vi "main.vi"() -> ()   [LabVIEW 2020]
doc: "This VI is used as the driver for the queue to work. It performs the operations in the queue."
uses:
  Typedef's/Data_Cluster.ctl
  Typedef's/Content_Level.ctl
  Typedef's/Bewarage_Out_Level.ctl
  Typedef's/Timer_Details.ctl
  Typedef's/Timings_Map.ctl
  Typedef's/Operation_Indication.ctl
  Typedef's/Low_Level_Indications.ctl
  Typedef's/Q_Operations.ctl
  <vilib>/Utility/error.llb/DialogType.ctl
  <vilib>/Utility/config.llb/Read Key (Boolean).vi
  <vilib>/Utility/config.llb/Read Key (I32).vi
  <vilib>/Utility/config.llb/Read Key (U32).vi
  <vilib>/Utility/config.llb/Write Key (U32).vi
  <vilib>/Utility/config.llb/Write Key (I32).vi
  <vilib>/Utility/config.llb/NI_LVConfig.lvlib
panel:
  in  "Error In":errorcluster
  in  "Power":bool
  out "Total Cups":u32
  out "Elapsed Time":i32
  out "Dispensing":bool
  out "Brewing":bool
  out "Grinding":bool
  out "Heating":bool
  out "Purging":bool
  in  "Dispenser":dbl(slide) min=-0.0 max=60.0 step=1.0 scale=0.0..60.0
  in  "Chamber":dbl(slide) min=-0.0 max=60.0 step=1.0 scale=0.0..60.0
  out "Low Milk":bool
  out "Low Bean":bool
  out "Low Water":bool
  out "Milk Level":i32(slide) min=0 max=100 step=1 scale=0.0..100.0
  out "Bean Level":i32(slide) min=0 max=100 step=1 scale=0.0..100.0
  out "Water Level":i32(slide) min=0 max=100 step=1 scale=0.0..100.0
  in  "Bewarage":i32(knob) min=0 max=2 step=1 scale=0.0..2.0
  in  "Carafe":bool
  in  "1 Cup":bool
  # "Description: \n-> Only after power run. Make the button press\nto make coffee"
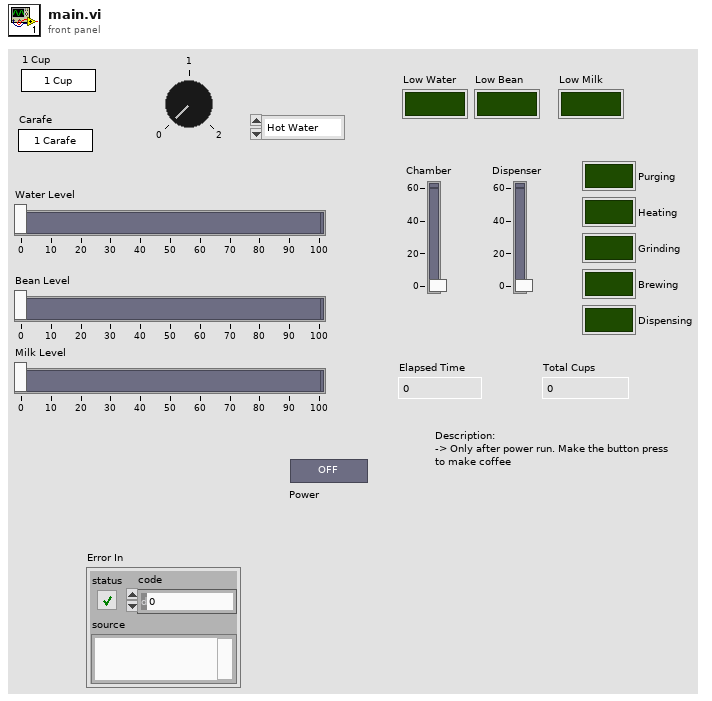
[diagram p1: front panel]
types:
  T1 = typedef "Q_Operations.ctl" = enum16{"Create Q", "Enqueue ", "Dequeue", "Enqueue N ele", "Enstack N ele", "Flush Q", "Destroy Q"}
  T2 = typedef "Data_Cluster.ctl" = cluster{"Cup":bool, "Bewarage":dbl, "Carafe":bool, "Power":bool, "Content Levels":T3, "Beware Out Level":T4, "Data File path":path, "Timer Operations":T5, "Cups Count":u32, "Bewarage Low Level":i32, "Timings Map":T6, "Sequence Array":string[], "Operation Indication":T7, "Bewarage Selection":string, "Low Level Indications":T8}
  T3 = typedef "Content_Level.ctl" = cluster{"Water Level":i32, "Bean Level":i32, "Milk Level":i32}
  T4 = typedef "Bewarage_Out_Level.ctl" = cluster{"Dispenser":dbl, "Chamber":dbl}
  T5 = typedef "Timer_Details.ctl" = cluster{"Set Time":dbl, "Prev Time":dbl, "Elapsed Time":dbl, "Start?":bool, "Paused?":bool}
  T6 = typedef "Timings_Map.ctl" = cluster{"Operation map":map{string, i32}, "Bevarage Timings":map{string, i32}}
  T7 = typedef "Operation_Indication.ctl" = cluster{"Heating":bool, "Grinding":bool, "Dispensing":bool, "Purging":bool, "Brewing":bool}
  T8 = typedef "Low_Level_Indications.ctl" = cluster{"Low Water":bool, "Low Milk":bool, "Low Bean":bool}
  T9 = typedef "NI_LVConfig.lvlib/Config Data RefNum.ctl" = refnum<k1>
  T10 = typedef "DialogType.ctl" = u16
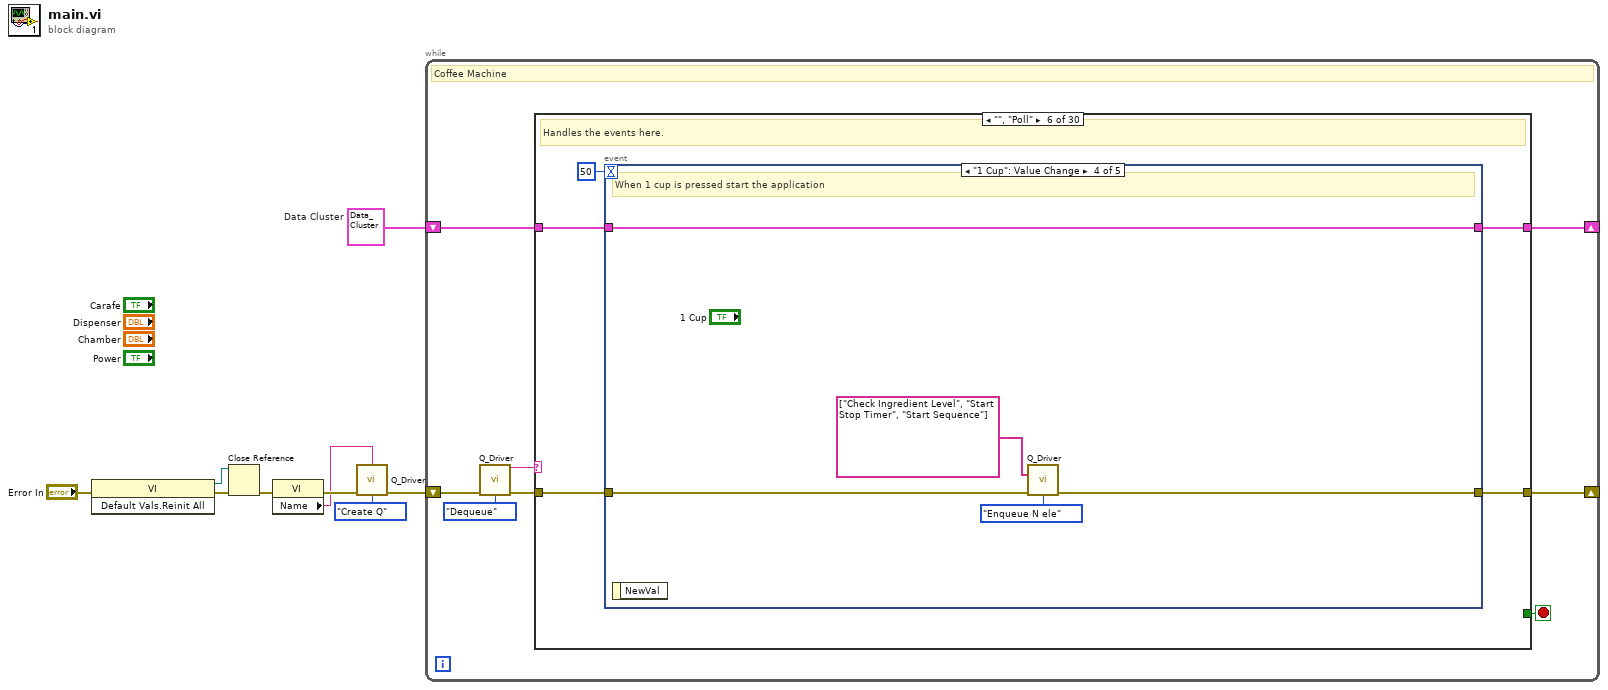
[diagram p0: block diagram]
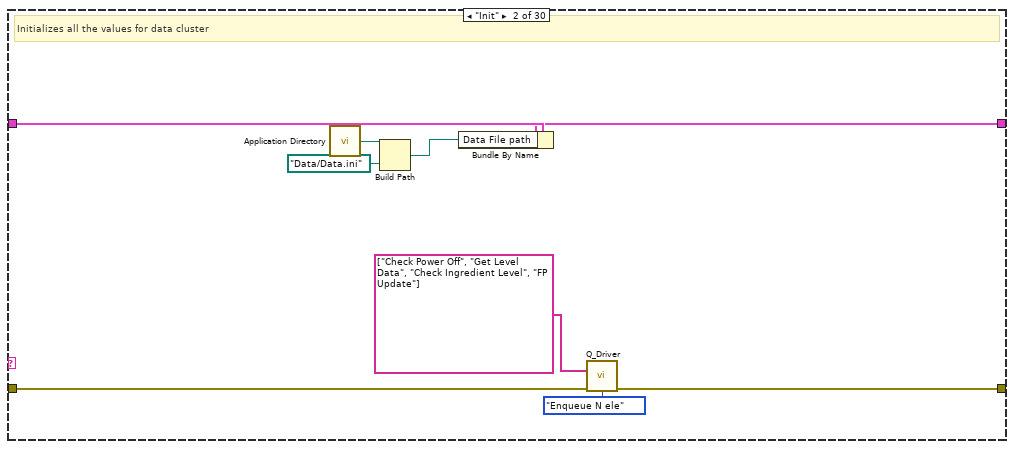
[diagram p3: hidden frame]
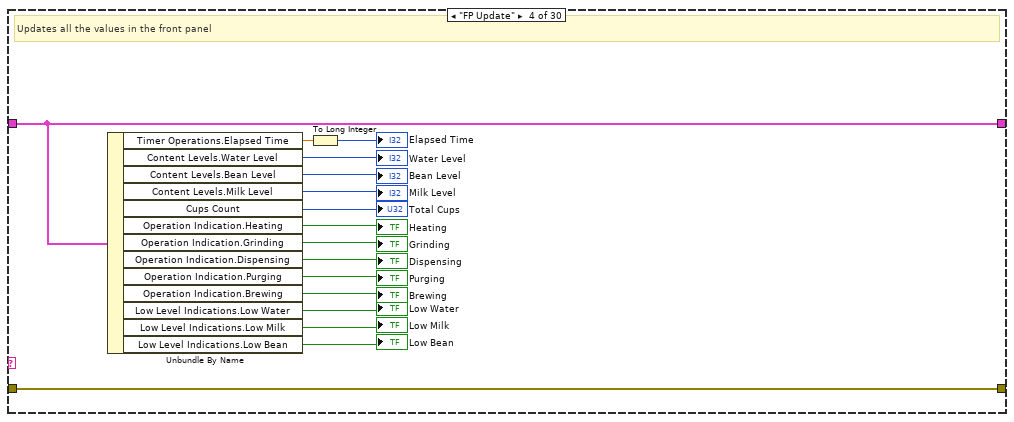
[diagram p5: hidden frame]
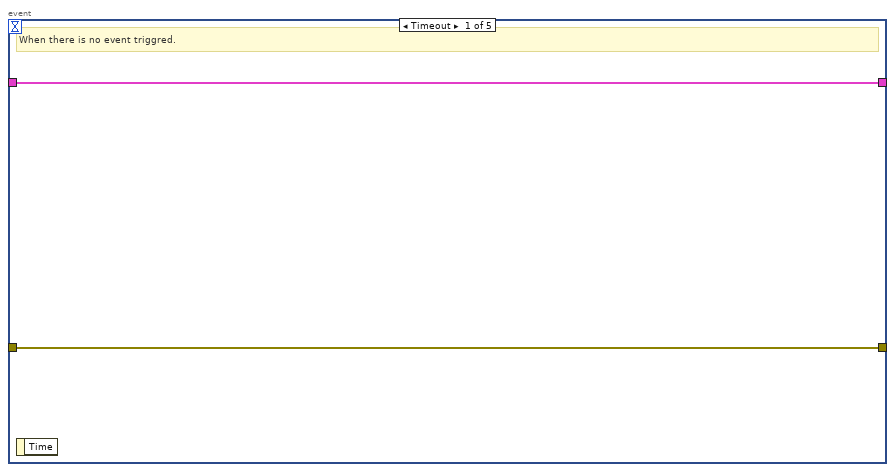
[diagram p7: hidden frame]
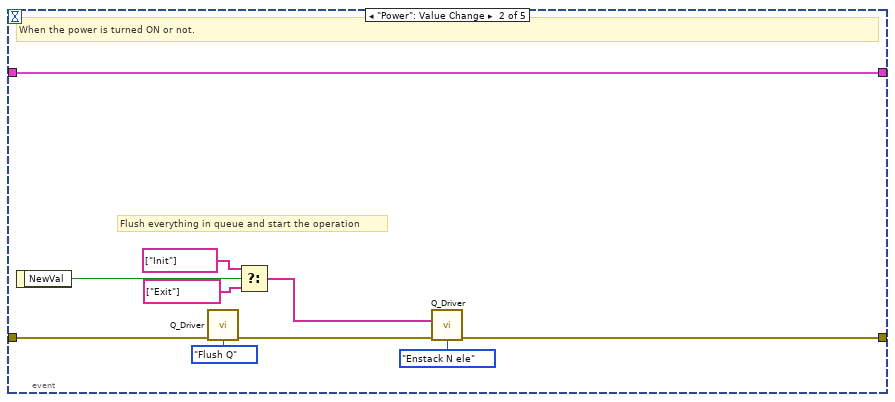
[diagram p8: hidden frame]
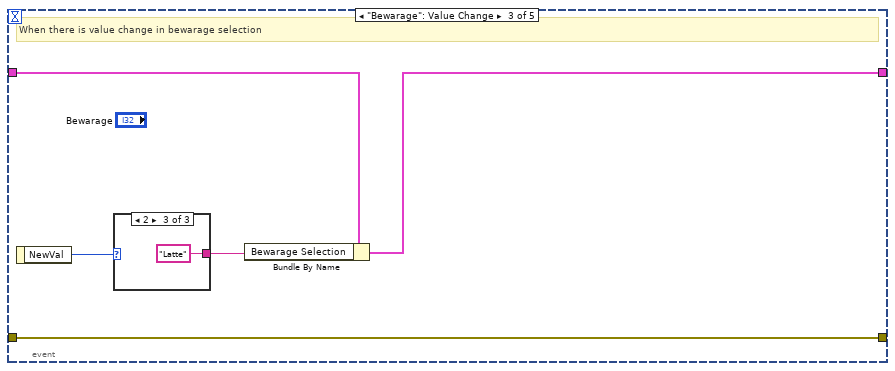
[diagram p9: hidden frame]
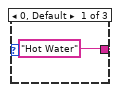
[diagram p10: hidden frame]
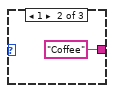
[diagram p11: hidden frame]
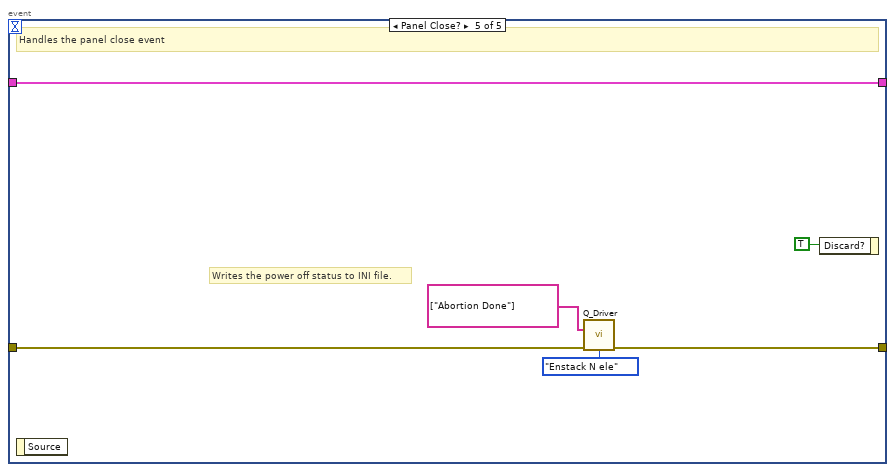
[diagram p12: hidden frame]
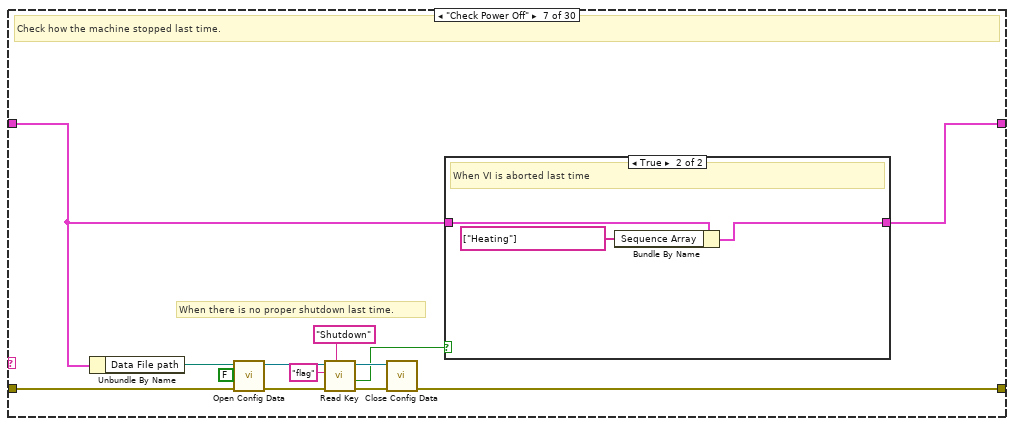
[diagram p13: hidden frame]
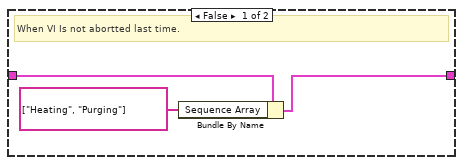
[diagram p14: hidden frame]
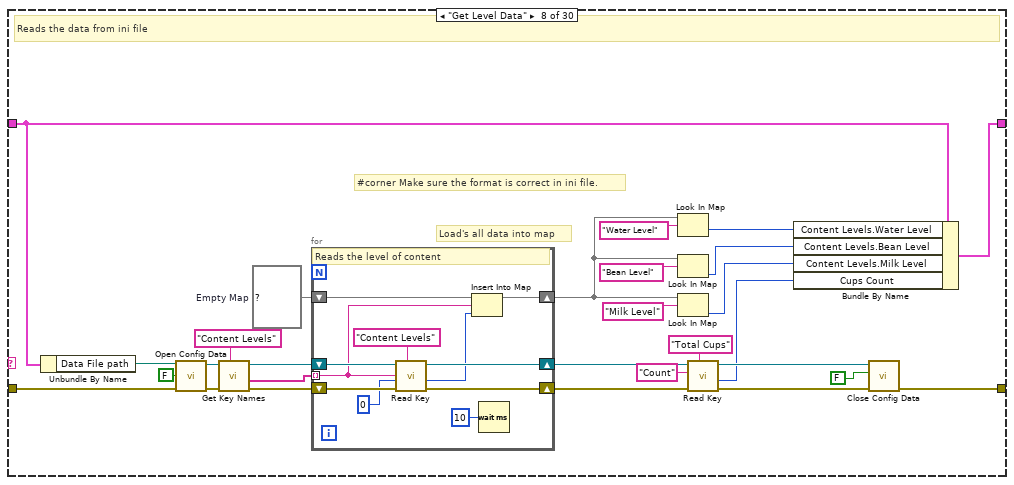
[diagram p15: hidden frame]
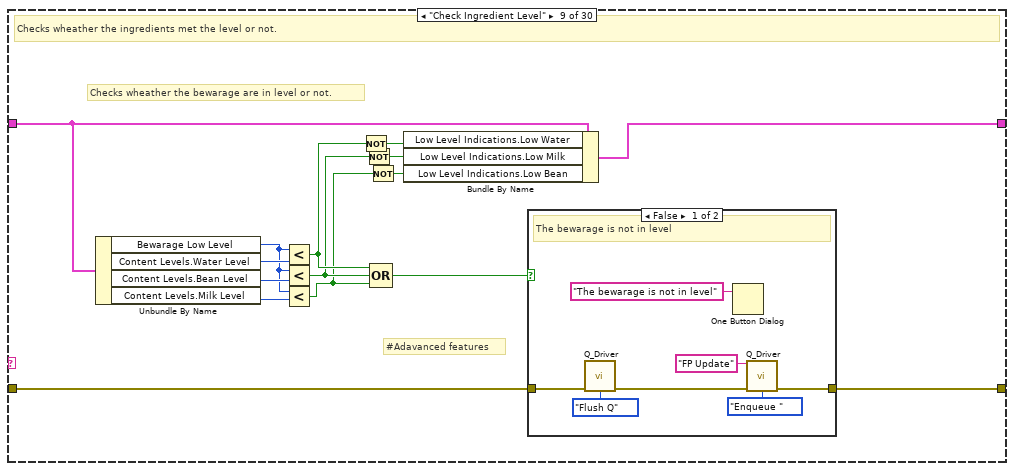
[diagram p16: hidden frame]
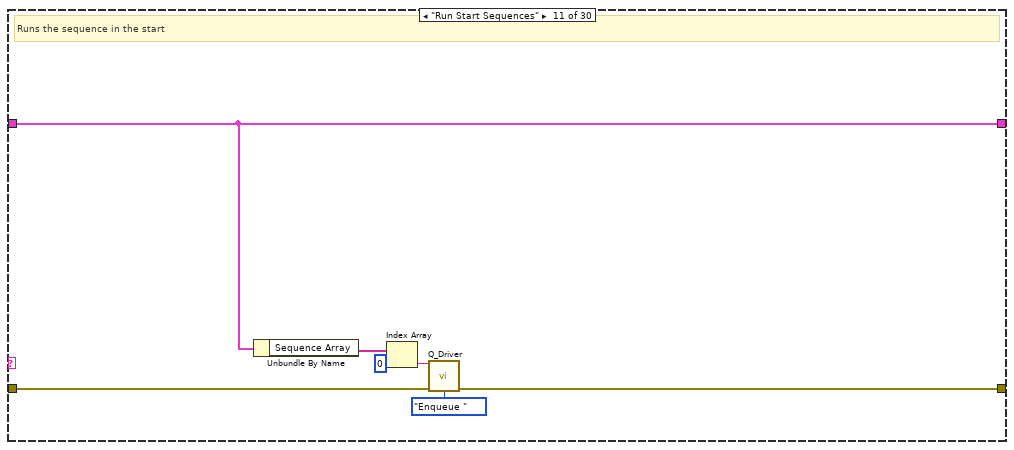
[diagram p19: hidden frame]
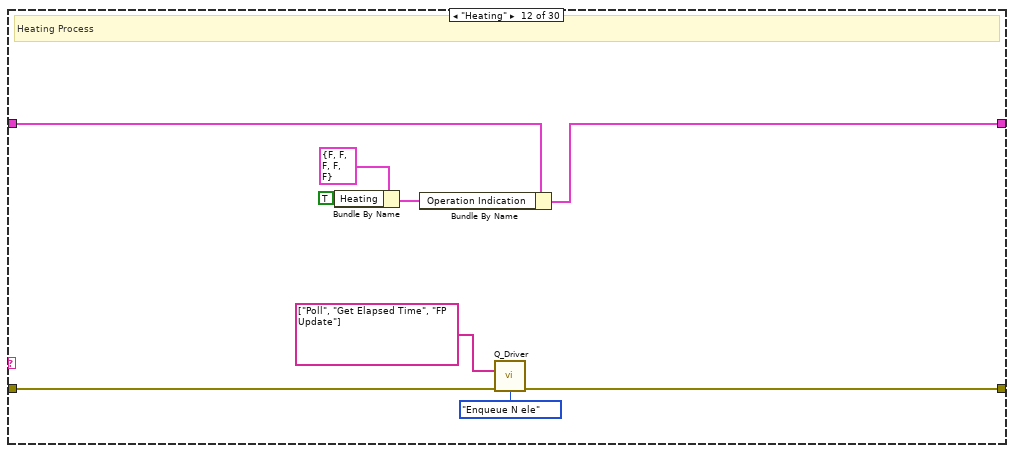
[diagram p20: hidden frame]
diagram:
  w4 = T2 {"Cup"=FALSE, "Bewarage"=0.0, "Carafe"=FALSE, "Power"=FALSE, "Content Levels"={"Water Level"=0, "Bean Level"=0, "Milk Level"=0}, "Beware Out Level"={"Dispenser"=0.0, "Chamber"=0.0}, "Data File path"=path "", "Timer Operations"={"Set Time"=0.0, "Prev Time"=0.0, "Elapsed Time"=0.0, "Start?"=FALSE, "Paused?"=FALSE}, "Cups Count"=0, "Bewarage Low Level"=30, "Timings Map"={"Operation map"={"Heating"=5, "Purging"=4}, "Bevarage Timings"={"Brewing"=4, "Dispensing"=5, "Grinding"=3}}, "Sequence Array"=[], "Operation Indication"={"Heating"=FALSE, "Grinding"=FALSE, "Dispensing"=FALSE, "Purging"=FALSE, "Brewing"=FALSE}, "Bewarage Selection"="Hot Water", "Low Level Indications"={"Low Water"=FALSE, "Low Milk"=FALSE, "Low Bean"=FALSE}}  # Data Cluster
  n1 = invoke class="VI" method="Default Vals.Reinit All"(error in="Error In") -> (reference out=w1:refnum<vi>, error out=w3:errorcluster)  [unwired: 2 in, 1 out]
  n2 = Close Reference(reference=w1, error in (no error)=w3) -> (error out=w2:errorcluster)
  n3 = property class="VI"(error in=w2) -> (error out=w6:errorcluster, "Name"=w5:string)  [unwired: 1 in, 1 out]
  n4 = call "Q_Driver.vi"("Q Name"=w5, "Error In"=w6, "Operations"=Q_Operations."Create Q") -> ("Error Out"=w8:errorcluster)  [unwired: 11 in, 1 out]
  n5 = while {
    shift-right: [w16] -> _
    shift-left: w8 -> [w17]
    shift-right: [w11] -> _
    shift-left: w4 -> [w12]
    stop <- w10 stop-if-true
    # "Coffee Machine"
    n6 = call "Q_Driver.vi"("Error In"=w17, "Operations"=Q_Operations."Dequeue") -> ("Dequeued Ele"=w13:string, "Error Out"=w15:errorcluster)  [unwired: 12 in]
    n7 = case shown="\"\", \"Poll\"" w13 {
      tunnel: w15 -> [w19 w27 w30 w46 w48 w53 w97 w131 w147 w167 w174 w183 w192 w194 w201 w240 w249 w250 w259 w276 w320 w322 w331 w342 w361 w367 w369 w375 w381 w383]
      tunnel: [w19 w26 w30 w46 w48 w52 w95 w128 w146 w167 w170 w181 w190 w194 w197 w239 w243 w251 w260 w271 w287 w322 w331 w333 w361 w364 w369 w372 w379 w383] -> w16
      tunnel: w12 -> [w18 w28 w29 w45 w47 w50 w86 w111 w157 w166 w173 w182 w191 w193 w199 w238 w248 w258 w263 w274 w315 w321 w329 w341 w360 w362 w368 w374 w378 w382]
      tunnel: [w18 w21 w29 w45 w47 w49 w85 w115 w151 w166 w173 w178 w187 w193 w198 w232 w247 w255 w264 w275 w305 w321 w330 w337 w360 w362 w368 w374 w378 w382] -> w11
      tunnel: [_ _ _ _ _ _ _ _ _ _ _ _ _ _ _ _ _ _ _ _ _ _ _ _ _ _ _ TRUE TRUE _] -> w10
      frame "/**** Initialization ****/" {
      }
      frame "Init" {
        # "Initializes all the values for data cluster"
        n8 = call <vilib>:"Application Directory.vi"() -> ("Application Directory"=w23:path)
        n9 = Build Path(base path=w23, name or relative path=path "Data/Data.ini") -> (appended path=w20:path)
        n10 = Bundle By Name(cluster=w28, "Data File path"=w20) -> (w21:T2)
        n11 = call "Q_Driver.vi"("States[]"=string[] ["Check Power Off", "Get Level Data", "Check Ingredient Level", "FP Update"], "Error In"=w27, "Operations"=Q_Operations."Enqueue N ele") -> ("Error Out"=w26:errorcluster)  [unwired: 11 in, 1 out]
      }
      frame "/***** FP Related ****/" {
      }
      frame "FP Update" {
        # "Updates all the values in the front panel"
        n12 = Unbundle By Name(w45) -> ("Timer Operations.Elapsed Time"=w35:dbl, "Content Levels.Water Level"=→"Water Level":i32, "Content Levels.Bean Level"=→"Bean Level":i32, "Content Levels.Milk Level"=→"Milk Level":i32, "Cups Count"=→"Total Cups":u32, "Operation Indication.Heating"=→"Heating":bool, "Operation Indication.Grinding"=→"Grinding":bool, "Operation Indication.Dispensing"=→"Dispensing":bool, "Operation Indication.Purging"=→"Purging":bool, "Operation Indication.Brewing"=→"Brewing":bool, "Low Level Indications.Low Water"=→"Low Water":bool, "Low Level Indications.Low Milk"=→"Low Milk":bool, "Low Level Indications.Low Bean"=→"Low Bean":bool)
        n13 = To Long Integer(number=w35) -> (32bit integer=→"Elapsed Time":i32)
      }
      frame "/***** Events and Functionalities *****/" {
      }
      frame "", "Poll" {
        # "Handles the events here."
        n14 = event shown="[3] \"1 Cup\": Value Change" {
          selector: _ -> [_ _ _ _ _]
          dyn-events: _ -> [_ _ _ _ _]
          timeout: 50 -> [_ _ _ _ _]
          tunnel: [w55 w60 w70 w76 w82] -> w52
          tunnel: w53 -> [w55 w65 w70 w78 w84]
          tunnel: [w54 w64 w67 w77 w79] -> w49
          tunnel: w50 -> [w54 w64 w69 w77 w79]
          event Timeout {
            # "When there is no event triggred."
            n15 = event-data() -> ()  [unwired: 1 in, 1 out]
          }
          event "Power": Value Change {
            # "Flush everything in queue and start the operation"
            # "When the power is turned ON or not."
            n16 = event-data() -> ("NewVal"=w63:bool)  [unwired: 1 in]
            n17 = call "Q_Driver.vi"("Error In"=w65, "Operations"=Q_Operations."Flush Q") -> ("Error Out"=w57:errorcluster)  [unwired: 12 in, 1 out]
            n18 = Select(t=string[] ["Init"], s=w63, f=string[] ["Exit"]) -> (s? t:f=w58:string[])
            n19 = call "Q_Driver.vi"("States[]"=w58, "Error In"=w57, "Operations"=Q_Operations."Enstack N ele") -> ("Error Out"=w60:errorcluster)  [unwired: 11 in, 1 out]
          }
          event "Bewarage": Value Change {
            # "When there is value change in bewarage selection"
            n20 = event-data() -> ("NewVal"=w68:i32)  [unwired: 1 in]
            n21 = case shown="2" w68 {
              tunnel: ["Hot Water" "Coffee" "Latte"] -> w66
              frame 0, Default {
              }
              frame 1 {
              }
              frame 2 {
              }
            }
            n22 = Bundle By Name(cluster=w69, "Bewarage Selection"=w66) -> (w67:T2)
          }
          event "1 Cup": Value Change {
            # "When 1 cup is pressed start the application"
            n23 = event-data() -> ()  [unwired: 1 in, 1 out]
            n24 = call "Q_Driver.vi"("States[]"=string[] ["Check Ingredient Level", "Start Stop Timer", "Start Sequence"], "Error In"=w78, "Operations"=Q_Operations."Enqueue N ele") -> ("Error Out"=w76:errorcluster)  [unwired: 11 in, 1 out]
          }
          event Panel Close? {
            # "Writes the power off status to INI file."
            # "Handles the panel close event"
            n25 = event-data() -> ()  [unwired: 1 in, 1 out]
            n26 = call "Q_Driver.vi"("States[]"=string[] ["Abortion Done"], "Error In"=w84, "Operations"=Q_Operations."Enstack N ele") -> ("Error Out"=w82:errorcluster)  [unwired: 11 in, 1 out]
            n27 = event-data("Discard?"=TRUE) -> ()  [unwired: 1 in, 1 out]
          }
        }
      }
      frame "Check Power Off" {
        # "When there is no proper shutdown last time."
        # "Check how the machine stopped last time."
        n28 = Unbundle By Name(w86) -> ("Data File path"=w88:path)
        n29 = call <vilib>:"Open Config Data.vi"("error in (no error)"=w97, "create file if necessary (T)"=FALSE, "configuration file path"=w88) -> ("error out"=w94:errorcluster, "refnum"=w93:T9)  [unwired: 6 in, 1 out]
        n30 = call-poly <vilib>:"Read Key.vi"("section"="Shutdown", "error in (no error)"=w94, "key"="flag", "refnum"=w93) -> ("error out"=w91:errorcluster, "value"=w87:bool, "refnum out"=w92:T9)  [unwired: 4 in, 1 out]
        n31 = call <vilib>:"Close Config Data.vi"("error in (no error)"=w91, "refnum"=w92) -> ("error out"=w95:errorcluster)  [unwired: 8 in, 1 out]
        n32 = case shown="True" w87 {
          tunnel: w86 -> [w100 w103]
          tunnel: [w99 w102] -> w85
          frame False {
            # "When VI Is not abortted last time."
            n33 = Bundle By Name(cluster=w100, "Sequence Array"=string[] ["Heating", "Purging"]) -> (w99:T2)
          }
          frame True {
            # "When VI is aborted last time"
            n34 = Bundle By Name(cluster=w103, "Sequence Array"=string[] ["Heating"]) -> (w102:T2)
          }
        }
      }
      frame "Get Level Data" {
        w121 = map{string, i32} {}  # Empty Map
        # "Load's all data into map"
        # "#corner Make sure the format is correct in ini file."
        # "Reads the data from ini file"
        n35 = Unbundle By Name(w111) -> ("Data File path"=w110:path)
        n36 = call <vilib>:"Open Config Data.vi"("error in (no error)"=w131, "create file if necessary (T)"=FALSE, "configuration file path"=w110) -> ("error out"=w129:errorcluster, "refnum"=w125:T9)  [unwired: 6 in, 1 out]
        n37 = call <vilib>:"Get Key Names.vi"("section"="Content Levels", "error in (no error)"=w129, "refnum"=w125) -> ("error out"=w126:errorcluster, "key names"=w123:string[], "refnum out"=w122:T9)  [unwired: 5 in, 1 out]
        n38 = for {
          shift-right: [w141] -> w124
          shift-left: w126 -> [w142]
          tunnel: w123 -> [w135] mode=indexing
          shift-right: [w138] -> w108
          shift-left: w122 -> [w139]
          shift-right: [w133] -> w116
          shift-left: w121 -> [w136]
          # "Reads the level of content"
          n39 = call-poly <vilib>:"Read Key.vi"("section"="Content Levels", "error in (no error)"=w142, "default value"=0, "key"=w135, "refnum"=w139) -> ("error out"=w141:errorcluster, "value"=w134:i32, "refnum out"=w138:T9)  [unwired: 3 in, 1 out]
          n40 = Insert Into Map(map in=w136, key=w135, value=w134) -> (map out=w133:map{string, i32})  [unwired: 2 out]
          n41 = Wait (ms)(milliseconds to wait=u32 10) -> ()  [unwired: 1 out]
        }
        n42 = Look In Map(map=w116, key="Water Level") -> (value=w114:i32)  [unwired: 1 in, 1 out]
        n43 = Look In Map(map=w116, key="Bean Level") -> (value=w113:i32)  [unwired: 1 in, 1 out]
        n44 = Look In Map(map=w116, key="Milk Level") -> (value=w112:i32)  [unwired: 1 in, 1 out]
        n45 = call-poly <vilib>:"Read Key.vi"("section"="Total Cups", "error in (no error)"=w124, "key"="Count", "refnum"=w108) -> ("error out"=w109:errorcluster, "value"=w106:u32, "refnum out"=w107:T9)  [unwired: 4 in, 1 out]
        n46 = Bundle By Name(cluster=w111, "Content Levels.Water Level"=w114, "Content Levels.Bean Level"=w113, "Content Levels.Milk Level"=w112, "Cups Count"=w106) -> (w115:T2)
        n47 = call <vilib>:"Close Config Data.vi"("error in (no error)"=w109, "write file if changed (T)"=FALSE, "refnum"=w107) -> ("error out"=w128:errorcluster)  [unwired: 7 in, 1 out]
      }
      frame "Check Ingredient Level" {
        # "#Adavanced features"
        # "Checks wheather the bewarage are in level or not."
        # "Checks wheather the ingredients met the level or not."
        n48 = Unbundle By Name(w157) -> ("Bewarage Low Level"=w153:i32, "Content Levels.Water Level"=w156:i32, "Content Levels.Bean Level"=w155:i32, "Content Levels.Milk Level"=w154:i32)
        n49 = Less?(x=w153, y=w156) -> (x < y?=w150:bool)
        n50 = Less?(x=w153, y=w155) -> (x < y?=w149:bool)
        n51 = Less?(x=w153, y=w154) -> (x < y?=w148:bool)
        n52 = Not(x=w150) -> (.not. x?=w145:bool)
        n53 = Not(x=w149) -> (.not. x?=w144:bool)
        n54 = Not(x=w148) -> (.not. x?=w143:bool)
        n55 = Compound Arithmetic op=OR(w150, w149, w148) -> (w152:bool)
        n56 = Bundle By Name(cluster=w157, "Low Level Indications.Low Water"=w145, "Low Level Indications.Low Milk"=w144, "Low Level Indications.Low Bean"=w143) -> (w151:T2)
        n57 = case shown="False" w152 {
          tunnel: w147 -> [w163 w165]
          tunnel: [w160 w165] -> w146
          frame False {
            # "The bewarage is not in level"
            n58 = call "Q_Driver.vi"("Error In"=w163, "Operations"=Q_Operations."Flush Q") -> ("Error Out"=w162:errorcluster)  [unwired: 12 in, 1 out]
            n59 = One Button Dialog(message="The bewarage is not in level") -> ()  [unwired: 1 in, 1 out]
            n60 = call "Q_Driver.vi"("State"="FP Update", "Error In"=w162, "Operations"=Q_Operations."Enqueue ") -> ("Error Out"=w160:errorcluster)  [unwired: 11 in, 1 out]
          }
          frame True {
            # "When they are in level"
          }
        }
      }
      frame "/***** Start Sequence Runners ****/" {
      }
      frame "Run Start Sequences" {
        # "Runs the sequence in the start"
        n61 = Unbundle By Name(w173) -> ("Sequence Array"=w172:string[])
        n62 = Index Array(array=w172, index=0) -> (element=w169:string)
        n63 = call "Q_Driver.vi"("State"=w169, "Error In"=w174, "Operations"=Q_Operations."Enqueue ") -> ("Error Out"=w170:errorcluster)  [unwired: 11 in, 1 out]
      }
      frame "Heating" {
        # "Heating Process"
        n64 = Bundle By Name(cluster=T7 {"Heating"=FALSE, "Grinding"=FALSE, "Dispensing"=FALSE, "Purging"=FALSE, "Brewing"=FALSE} ("Operation Indication"), "Heating"=TRUE) -> (w177:T7)
        n65 = Bundle By Name(cluster=w182, "Operation Indication"=w177) -> (w178:T2)
        n66 = call "Q_Driver.vi"("States[]"=string[] ["Poll", "Get Elapsed Time", "FP Update"], "Error In"=w183, "Operations"=Q_Operations."Enqueue N ele") -> ("Error Out"=w181:errorcluster)  [unwired: 11 in, 1 out]
      }
      frame "Purging" {
        # "Purging process to be done"
        n67 = Bundle By Name(cluster=T7 {"Heating"=FALSE, "Grinding"=FALSE, "Dispensing"=FALSE, "Purging"=FALSE, "Brewing"=FALSE} ("Operation Indication"), "Purging"=TRUE) -> (w184:T7)
        n68 = Bundle By Name(cluster=w191, "Operation Indication"=w184) -> (w187:T2)
        n69 = call "Q_Driver.vi"("States[]"=string[] ["Poll", "Get Elapsed Time", "FP Update"], "Error In"=w192, "Operations"=Q_Operations."Enqueue N ele") -> ("Error Out"=w190:errorcluster)  [unwired: 11 in, 1 out]
      }
      frame "/**** Sequence Runners ****/" {
        # "States to run the sequences."
      }
      frame "Start Sequence" {
        # "Starts the sequence by updating things into tthe array"
        n70 = Unbundle By Name(w199) -> ("Bewarage Selection"=w200:string)
        n71 = case shown="\"Latte\"" w200 {
          tunnel: w199 -> [w206 w215 w227 w229]
          tunnel: [w202 w208 w217 w229] -> w198
          frame "Hot Water" {
            n72 = Unbundle By Name(w206) -> ("Content Levels.Water Level"=w205:i32)
            n73 = Subtract(x=w205, y=5) -> (x-y=w204:i32)
            n74 = Bundle By Name(cluster=w206, "Sequence Array"=string[] ["Dispensing"], "Content Levels.Water Level"=w204) -> (w202:T2)
          }
          frame "Coffee" {
            n75 = Unbundle By Name(w215) -> ("Content Levels.Water Level"=w213:i32, "Content Levels.Water Level"=w210:i32)
            n76 = Subtract(x=w213, y=5) -> (x-y=w211:i32)
            n77 = Subtract(x=w210, y=5) -> (x-y=w209:i32)
            n78 = Bundle By Name(cluster=w215, "Sequence Array"=string[] ["Grinding", "Brewing", "Dispensing"], "Content Levels.Bean Level"=w211, "Content Levels.Water Level"=w209) -> (w208:T2)
          }
          frame "Latte" {
            n79 = Unbundle By Name(w227) -> ("Content Levels.Water Level"=w225:i32, "Content Levels.Bean Level"=w223:i32, "Content Levels.Milk Level"=w221:i32)
            n80 = Subtract(x=w225, y=5) -> (x-y=w220:i32)
            n81 = Subtract(x=w223, y=5) -> (x-y=w219:i32)
            n82 = Subtract(x=w221, y=5) -> (x-y=w218:i32)
            n83 = Bundle By Name(cluster=w227, "Sequence Array"=string[] ["Grinding", "Brewing", "Dispensing"], "Content Levels.Water Level"=w220, "Content Levels.Bean Level"=w219, "Content Levels.Milk Level"=w218) -> (w217:T2)
          }
          frame Default {
          }
        }
        n84 = call "Q_Driver.vi"("State"="Run Sequence", "Error In"=w201, "Operations"=Q_Operations."Enqueue ") -> ("Error Out"=w197:errorcluster)  [unwired: 11 in, 1 out]
      }
      frame "Run Sequence" {
        # "Takes the first element in sequence array and run's for that particular time."
        # "Runs the sequence"
        n85 = Unbundle By Name(w238) -> ("Timings Map.Bevarage Timings"=w233:map{string, i32}, "Sequence Array"=w237:string[])
        n86 = Index Array(array=w237, index=0) -> (element=w234:string)
        n87 = call "Q_Driver.vi"("State"=w234, "Error In"=w240, "Operations"=Q_Operations."Enqueue ") -> ("Error Out"=w239:errorcluster)  [unwired: 11 in, 1 out]
        n88 = Look In Map(map=w233, key=w234) -> (value=w231:i32)  [unwired: 1 in, 1 out]
        n89 = To Double Precision Float(number=w231) -> (double precision float=w230:dbl)
        n90 = Bundle By Name(cluster=w238, "Timer Operations.Set Time"=w230) -> (w232:T2)
      }
      frame "Grinding" {
        n91 = Bundle By Name(cluster=T7 {"Heating"=FALSE, "Grinding"=FALSE, "Dispensing"=FALSE, "Purging"=FALSE, "Brewing"=FALSE} ("Operation Indication"), "Grinding"=TRUE) -> (w244:T7)
        n92 = Bundle By Name(cluster=w248, "Operation Indication"=w244) -> (w247:T2)
        n93 = call "Q_Driver.vi"("States[]"=string[] ["FP Update", "Get Elapsed Time", "Poll"], "Error In"=w249, "Operations"=Q_Operations."Enqueue N ele") -> ("Error Out"=w243:errorcluster)  [unwired: 11 in, 1 out]
      }
      frame "Brewing" {
        n94 = Bundle By Name(cluster=T7 {"Heating"=FALSE, "Grinding"=FALSE, "Dispensing"=FALSE, "Purging"=FALSE, "Brewing"=FALSE} ("Operation Indication"), "Brewing"=TRUE ("Grinding")) -> (w254:T7)
        n95 = Bundle By Name(cluster=w258, "Operation Indication"=w254) -> (w255:T2)
        n96 = call "Q_Driver.vi"("States[]"=string[] ["FP Update", "Get Elapsed Time", "Poll"], "Error In"=w250, "Operations"=Q_Operations."Enqueue N ele") -> ("Error Out"=w251:errorcluster)  [unwired: 11 in, 1 out]
      }
      frame "Dispensing" {
        n97 = Bundle By Name(cluster=T7 {"Heating"=FALSE, "Grinding"=FALSE, "Dispensing"=FALSE, "Purging"=FALSE, "Brewing"=FALSE} ("Operation Indication"), "Dispensing"=TRUE ("Grinding")) -> (w265:T7)
        n98 = Bundle By Name(cluster=w263, "Operation Indication"=w265) -> (w264:T2)
        n99 = call "Q_Driver.vi"("States[]"=string[] ["FP Update", "Get Elapsed Time", "Poll"], "Error In"=w259, "Operations"=Q_Operations."Enqueue N ele") -> ("Error Out"=w260:errorcluster)  [unwired: 11 in, 1 out]
      }
      frame "Go To Next Sequence" {
        # "Once one sequence is finished run's the next sequence."
        n100 = Unbundle By Name(w274) -> ("Sequence Array"=w273:string[])
        n101 = Delete From Array(array=w273, index=0) -> (array with subset deleted=w270:string[])  [unwired: 1 in, 1 out]
        n102 = Empty Array?(array=w270) -> (empty?=w269:bool)
        n103 = case shown="True" w269 {
          tunnel: w276 -> [w280 w284]
          tunnel: [w279 w283] -> w271
          frame False {
            # "Operate next seq"
            n104 = call "Q_Driver.vi"("State"="Run Sequence", "Error In"=w280, "Operations"=Q_Operations."Enqueue ") -> ("Error Out"=w279:errorcluster)  [unwired: 11 in, 1 out]
          }
          frame True {
            # "Operation finished"
            n105 = call "Q_Driver.vi"("State"="Operation Finished", "Error In"=w284, "Operations"=Q_Operations."Enqueue ") -> ("Error Out"=w283:errorcluster)  [unwired: 11 in, 1 out]
          }
        }
        n106 = Bundle By Name(cluster=w274, "Sequence Array"=w270, "Timer Operations.Elapsed Time"=0.0) -> (w275:T2)
      }
      frame "Operation Finished" {
        w294 = "Content Levels" ("section")
        # "Finished running operation"
        n107 = Unbundle By Name(w315) -> ("Cups Count"=w314:u32, "Data File path"=w312:path)
        n108 = call "Q_Driver.vi"("States[]"=string[] ["FP Update"], "Error In"=w320, "Operations"=Q_Operations."Enqueue N ele") -> ("Error Out"=w318:errorcluster)  [unwired: 11 in, 1 out]
        n109 = Increment(x=w314) -> (x+1=w307:u32)
        n110 = Bundle By Name(cluster=w315, "Operation Indication"=T7 {"Heating"=FALSE, "Grinding"=FALSE, "Dispensing"=FALSE, "Purging"=FALSE, "Brewing"=FALSE}, "Cups Count"=w307) -> (w305:T2)
        n111 = call <vilib>:"Open Config Data.vi"("error in (no error)"=w318, "configuration file path"=w312) -> ("error out"=w313:errorcluster, "refnum"=w310:T9)  [unwired: 7 in, 1 out]
        n112 = Unbundle By Name(w305) -> ("Content Levels.Water Level"=w303:i32, "Content Levels.Bean Level"=w299:i32, "Content Levels.Milk Level"=w292:i32)
        n113 = call-poly <vilib>:"Write Key.vi"("section"="Total Cups", "error in (no error)"=w313, "value"=w307, "key"="count", "refnum"=w310) -> ("error out"=w311:errorcluster, "refnum out"=w297:T9)  [unwired: 4 in, 1 out]
        n114 = call-poly <vilib>:"Write Key.vi"("section"=w294, "error in (no error)"=w311, "value"=w303, "key"="Water Level", "refnum"=w297) -> ("error out"=w301:errorcluster, "refnum out"=w296:T9)  [unwired: 4 in, 1 out]
        n115 = call-poly <vilib>:"Write Key.vi"("section"=w294, "error in (no error)"=w301, "value"=w299, "key"="Bean Level", "refnum"=w296) -> ("error out"=w300:errorcluster, "refnum out"=w295:T9)  [unwired: 4 in, 1 out]
        n116 = call-poly <vilib>:"Write Key.vi"("section"=w294, "error in (no error)"=w300, "value"=w292, "key"="Milk Level", "refnum"=w295) -> ("error out"=w298:errorcluster, "refnum out"=w291:T9)  [unwired: 4 in, 1 out]
        n117 = call <vilib>:"Close Config Data.vi"("error in (no error)"=w298, "write file if changed (T)"=TRUE, "refnum"=w291) -> ("error out"=w306:errorcluster)  [unwired: 7 in, 1 out]
        n118 = call "Q_Driver.vi"("Error In"=w306, "Operations"=Q_Operations."Flush Q") -> ("Error Out"=w289:errorcluster)  [unwired: 12 in, 1 out]
        n119 = call "Q_Driver.vi"("State"="Init", "Error In"=w289, "Operations"=Q_Operations."Enqueue ") -> ("Error Out"=w287:errorcluster)  [unwired: 11 in, 1 out]
      }
      frame "/**** Timer Operations ****/" {
      }
      frame "Start Stop Timer" {
        # "Starts the timer"
        n120 = Unbundle By Name(w329) -> ("Timer Operations.Start?"=w328:bool)
        n121 = Get Date/Time In Seconds() -> (seconds since 1Jan1904=w326:timestamp)
        n122 = To Double Precision Float(number=w326) -> (double precision float=w324:dbl)
        n123 = Not(x=w328) -> (.not. x?=w327:bool)
        n124 = Bundle By Name(cluster=w329, "Timer Operations.Start?"=w327, "Timer Operations.Set Time"=0.0, "Timer Operations.Prev Time"=w324, "Timer Operations.Paused?"=FALSE) -> (w330:T2)
      }
      frame "Get Elapsed Time" {
        # "When set point is reached"
        # "Get's the elapsed time between the runs."
        n125 = Unbundle By Name(w341) -> ("Timer Operations.Paused?"=w340:bool, "Timer Operations.Prev Time"=w339:dbl, "Timer Operations.Elapsed Time"=w338:dbl, "Timer Operations.Set Time"=w335:dbl)
        n126 = case shown="False" w340 {
          tunnel: w339 -> [w354 _]
          tunnel: w338 -> [w352 w357]
          tunnel: [w355 w358] -> w336
          tunnel: [w353 w357] -> w334
          frame False {
            # "When timer is paused"
            n127 = Get Date/Time In Seconds() -> (seconds since 1Jan1904=w356:timestamp)
            n128 = To Double Precision Float(number=w356) -> (double precision float=w355:dbl)
            n129 = Subtract(x=w355, y=w354) -> (x-y=w351:dbl)
            n130 = Add(x=w351, y=w352) -> (x+y=w353:dbl)
          }
          frame True {
            # "When timer is not paused"
            n131 = Get Date/Time In Seconds() -> (seconds since 1Jan1904=w359:timestamp)
            n132 = To Double Precision Float(number=w359) -> (double precision float=w358:dbl)
          }
        }
        n133 = Greater?(x=w334, y=w335) -> (0:w332:bool)
        n134 = case shown="False" w332 {
          tunnel: w342 -> [w346 w350]
          tunnel: [w345 w349] -> w333
          frame False {
            # "Doesn't reached setpoint"
            n135 = call "Q_Driver.vi"("States[]"=string[] ["Run Sequence"], "Error In"=w346, "Operations"=Q_Operations."Enqueue N ele") -> ("Error Out"=w345:errorcluster)  [unwired: 11 in, 1 out]
          }
          frame True {
            # "REached set point"
            n136 = call "Q_Driver.vi"("States[]"=string[] ["Go To Next Sequence"], "Error In"=w350, "Operations"=Q_Operations."Enqueue N ele") -> ("Error Out"=w349:errorcluster)  [unwired: 11 in, 1 out]
          }
        }
        n137 = Bundle By Name(cluster=w341, "Timer Operations.Prev Time"=w336, "Timer Operations.Elapsed Time"=w334) -> (w337:T2)
      }
      frame "/**** Errors *****/" {
      }
      frame "Error" {
        w365 = T10 2 items=["no dialog", "OK message", "continue or stop message", "OK message + warnings", "continue/stop + warnings"] ("type of dialog (OK msg:1)")
        # "Just pop up the errror"
        # "Handle the error's here"
        n138 = call <vilib>:"Simple Error Handler.vi"("type of dialog (OK msg:1)"=w365, "error in (no error)"=w367) -> ("code out"=w363:i32, "error out"=w366:errorcluster)  [unwired: 3 in, 3 out]
        n139 = call <vilib>:"Clear Errors.vi"("error in (no error)"=w366, "specific error code to clear (0: all)"=w363) -> ("error out"=w364:errorcluster)  [unwired: 4 in, 1 out]
      }
      frame "/ ***** Exit ***** /" {
      }
      frame "Abortion Done" {
        # "Aborting the VI has done. Write the data into ini file"
        n140 = Unbundle By Name(w374) -> ("Data File path"=w373:path)
        n141 = call "Write_Power_Off_Status.vi"("Data File path"=w373, "Value"=TRUE, "error in (no error)"=w375) -> ("error out"=w372:errorcluster)  [unwired: 12 in]
      }
      frame "Exit" {
        # "Writes the status of power off in the ini file."
        # "Handles operations during exit"
        n142 = Unbundle By Name(w378) -> ("Data File path"=w377:path)
        n143 = call "Write_Power_Off_Status.vi"("Data File path"=w377, "Value"=FALSE, "error in (no error)"=w381) -> ("error out"=w379:errorcluster)  [unwired: 12 in]
      }
      frame "Developer Error", Default {
        # "Mistakes done by developer"
      }
    }
  }
